vi "Configure Bandwidth Part.vi"(0 "VISA resource name":refnum<visa-resource-name>, 1 "Subcarrier Spacing (120 kHz)":T2=1 items=["60 kHz", "120 kHz"], 2 "No Of RBs (66)":i32=66, 5 "Instance (1)":T5=1, 7 "Carrier Component (1)":T4=1, 9 "Bandwidth Part (BWP0)":T3 items=["BWP0"], 11 "error in (no error)":errorcluster, 12 "Cyclic Prefix (Normal)":T1 items=["Normal"], 13 "Start RB (0)":i32) -> (4 "VISA resource name out":refnum<visa-resource-name>, 15 "error out":errorcluster)   [LabVIEW 2015, in "Rohde&Schwarz CMXP NR FR2 Measurement.lvlib"]
doc: "Configures basic properties of the <BWP> on carrier <CC>.\n\nAttribute:\nRSCMXPNRFR2M_ATTR_BANDWIDTH_PART\n\nRemote-control command:\nCONFigure:NRMMw:MEAS<i>[:CC<no>]:BWPart"
uses:
  <instrlib>/Rohde&Schwarz CMXP NR FR2 Measurement/Rohde&Schwarz CMXP NR FR2 Measurement.lvlib
  <instrlib>/Rohde&Schwarz CMXP NR FR2 Measurement/Private/_Instance.ctl
  <instrlib>/Rohde&Schwarz CMXP NR FR2 Measurement/Private/_Carrier Component.ctl
  <instrlib>/Rohde&Schwarz CMXP NR FR2 Measurement/Private/_Bandwidth Part.ctl
  <instrlib>/Rohde&Schwarz CMXP NR FR2 Measurement/Private/_Subcarrier Spacing.ctl
  <instrlib>/Rohde&Schwarz CMXP NR FR2 Measurement/Private/_Cyclic Prefix.ctl
  <instrlib>/Rohde&Schwarz CMXP NR FR2 Measurement/Private/rsidr_core.llb/rsidr_core.lvlib
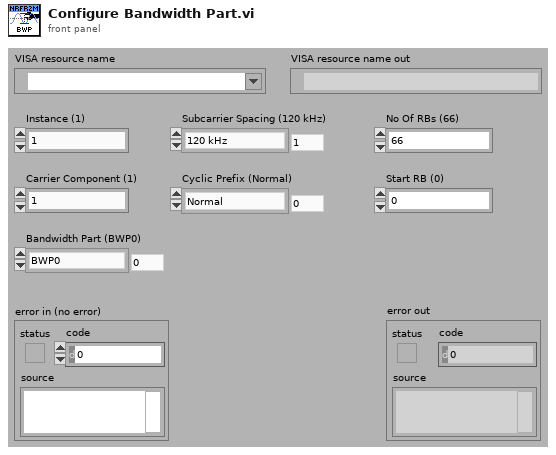
[diagram p1: front panel]
types:
  T1 = typedef "Rohde&Schwarz CMXP NR FR2 Measurement.lvlib/_Cyclic Prefix.ctl" = i32
  T2 = typedef "Rohde&Schwarz CMXP NR FR2 Measurement.lvlib/_Subcarrier Spacing.ctl" = i32
  T3 = typedef "Rohde&Schwarz CMXP NR FR2 Measurement.lvlib/_Bandwidth Part.ctl" = i32
  T4 = typedef "Rohde&Schwarz CMXP NR FR2 Measurement.lvlib/_Carrier Component.ctl" = i32
  T5 = typedef "Rohde&Schwarz CMXP NR FR2 Measurement.lvlib/_Instance.ctl" = i32
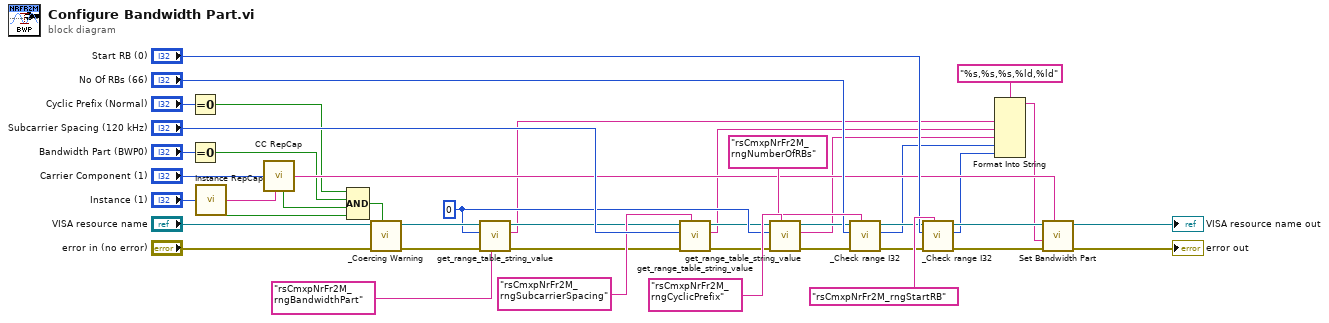
[diagram p0: block diagram]
diagram:
  w27 = 0
  n1 = Equal To 0?(x="Cyclic Prefix (Normal)") -> (x = 0?=w4:bool)
  n2 = Equal To 0?(x="Bandwidth Part (BWP0)") -> (x = 0?=w5:bool)
  n3 = call <instrlib>:"Instance RepCap.vi"("Instance In"="Instance (1)") -> ("In Range?"=w39:bool, "RepCap Identifier Out"=w2:string)  [unwired: 1 in]
  n4 = call <instrlib>:"CC RepCap.vi"("CC In"="Carrier Component (1)", "RepCap String In (\"\")"=w2) -> ("In Range?"=w38:bool, "RepCap Identifier Out"=w13:string)
  n5 = Compound Arithmetic op=AND(w4, w5, w38, w39) -> (w41:bool)
  n6 = call <instrlib>:"_Coercing Warning.vi"("In Range?"=w41, "error in (no error)"="error in (no error)", "VISA resource name"="VISA resource name") -> ("error out"=w34:errorcluster, "VISA resource name out"=w31:refnum<visa-resource-name>)  [unwired: 7 in]
  n7 = call <instrlib>:"get_range_table_string_value.vi"("Range Table ID in"="rsCmxpNrFr2M_rngBandwidthPart", "error in"=w34, "I32 input"=w27, "VISA resource name"=w31) -> ("error out"=w29:errorcluster, "String Value out"=w10:string, "VISA resource name out"=w30:refnum<visa-resource-name>)  [unwired: 5 in]
  n8 = call <instrlib>:"get_range_table_string_value.vi"("Range Table ID in"="rsCmxpNrFr2M_rngSubcarrierSpacing", "error in"=w29, "I32 input"="Subcarrier Spacing (120 kHz)", "VISA resource name"=w30) -> ("error out"=w26:errorcluster, "String Value out"=w9:string, "VISA resource name out"=w25:refnum<visa-resource-name>)  [unwired: 5 in]
  n9 = call <instrlib>:"get_range_table_string_value.vi"("Range Table ID in"="rsCmxpNrFr2M_rngCyclicPrefix", "error in"=w26, "I32 input"=w27, "VISA resource name"=w25) -> ("error out"=w21:errorcluster, "String Value out"=w8:string, "VISA resource name out"=w22:refnum<visa-resource-name>)  [unwired: 5 in]
  n10 = call <instrlib>:"_Check range I32.vi"("Range Table Identifier"="rsCmxpNrFr2M_rngNumberOfRBs", "error in (no error)"=w21, "I32 Value In"="No Of RBs (66)", "VISA resource name"=w22) -> ("error out"=w18:errorcluster, "I32 Value Out"=w7:i32, "VISA resource name out"=w17:refnum<visa-resource-name>)  [unwired: 5 in]
  n11 = call <instrlib>:"_Check range I32.vi"("Range Table Identifier"="rsCmxpNrFr2M_rngStartRB", "error in (no error)"=w18, "I32 Value In"="Start RB (0)", "VISA resource name"=w17) -> ("error out"=w15:errorcluster, "I32 Value Out"=w6:i32, "VISA resource name out"=w16:refnum<visa-resource-name>)  [unwired: 5 in]
  n12 = Format Into String(format string="%s,%s,%s,%ld,%ld", w10, w9, w8, w7, w6) -> (resulting string=w1:string)  [unwired: 2 in, 1 out]
  n13 = call "Set Bandwidth Part"("Repeated Capabilities"=w13, "error in (no error)"=w15, "Bandwidth Part ()"=w1, "instrument handle"=w16) -> ("error out"=→"error out":errorcluster, "instrument handle out"=→"VISA resource name out":refnum<visa-resource-name>)  [unwired: 6 in]
